vi "MSSQL_Select.vi"(0 "connection reference":T1, 1 "列名数组":string[](array[string]), 3 "排序条件":string, 5 "表名":string, 9 "查询行数":i32, 11 "异常输入":errorcluster, 12 "查询条件":string) -> (4 "connection reference 2":T1, 6 "变体转换后数据":string[][](array[string]), 8 "完整数据":variant[][](array[variant]), 10 "拼接后的sql语句":string, 14 "操作结果":bool, 15 "异常输出":errorcluster)   [LabVIEW 2018]
uses:
  <vilib>/addons/database/Connection.llb/Conn ObjectReference.ctl
  <vilib>/addons/database/Connection.llb/Conn Execute.vi
  <vilib>/addons/database/Recordset.llb/Rec Fetch Recordset Data (R).vi
  <vilib>/addons/database/Recordset.llb/Rec Destroy - Connection.vi
  <vilib>/addons/database/NI_Database_API.lvlib
panel:
  # "select操作\nselect * from tbl_name where 条件 order by \nselect 列1，列2，列3 from tbl_name where 条件 order by \nselect操作\nselect top(1) * from tbl_name where 条件 order by \nselect top(1) 列1，列2，列3 from tbl_name where 条件 order by"
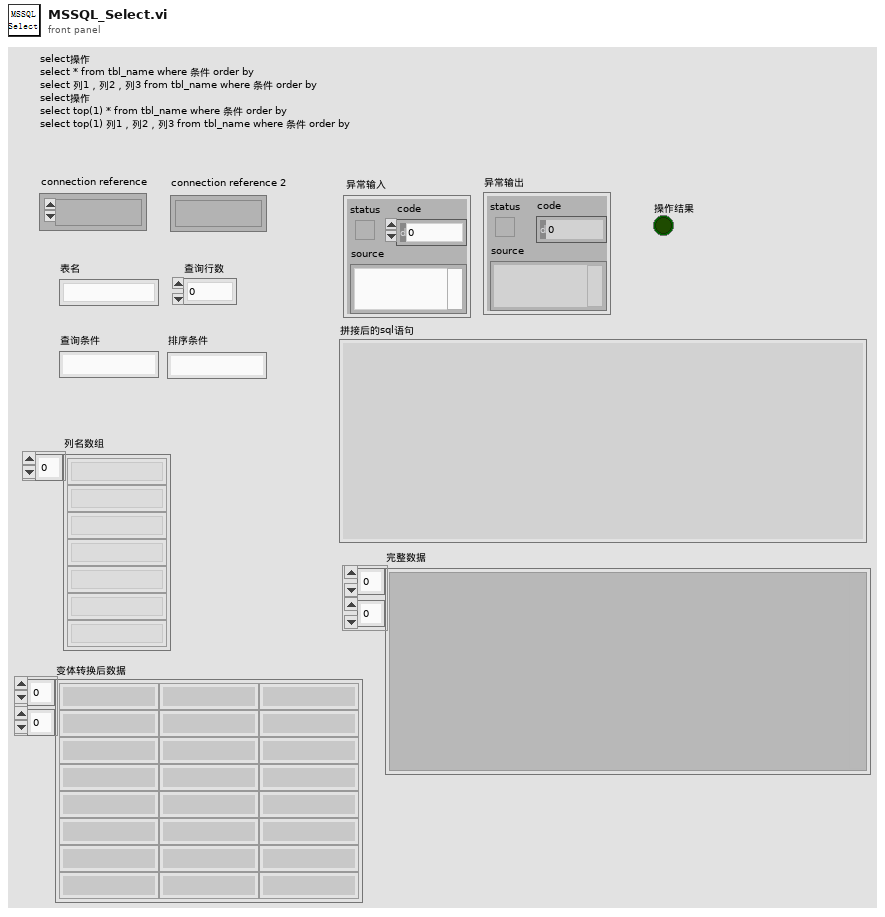
[diagram p1: front panel]
types:
  T1 = typedef "NI_Database_API.lvlib/Conn ObjectReference.ctl" = refnum<k1>
  T2 = typedef "NI_Database_API.lvlib/Rec ObjectReference.ctl" = refnum<k1>
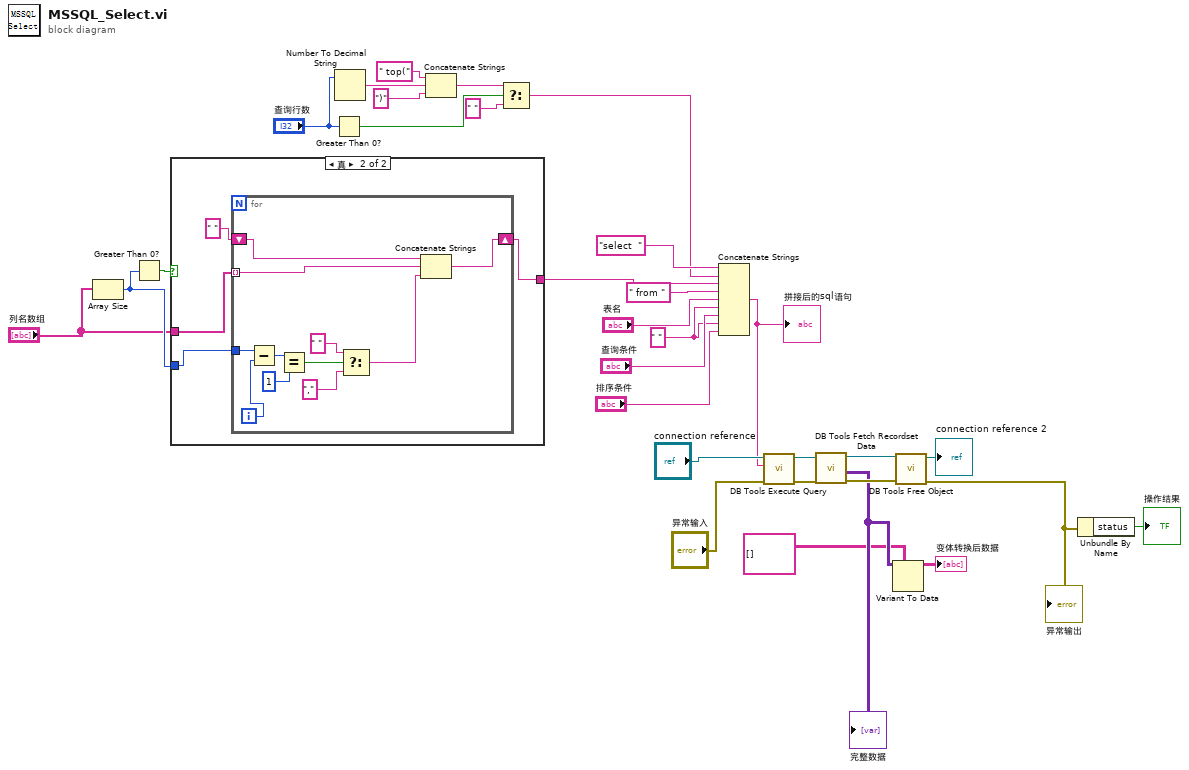
[diagram p0: block diagram]
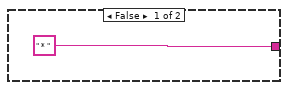
[diagram p2: hidden frame]
diagram:
  w9 = " " ("字符串")
  n1 = Array Size(array="列名数组") -> (size(s)=w29:i32)
  n2 = Greater Than 0?(x=w29) -> (x > 0?=w30:bool)
  n3 = case shown="真" w30 {
    tunnel: [" * " w33] -> w28
    tunnel: w29 -> [_ w36]
    tunnel: "列名数组" -> [_ w35]
    frame False {
    }
    frame True {
      n4 = for {
        tunnel: w35 -> [w46] mode=indexing
        shift-right: [w45] -> w33
        shift-left: " " -> [w47]
        tunnel: w36 -> [w37]
        i -> [w44]
        n5 = Subtract(x=w37, y=w44) -> (x-y=w43:i32)
        n6 = Equal?(x=w43, y=1) -> (x = y?=w41:bool)
        n7 = Select(t=" " ("字符串"), s=w41, f=",") -> (s? t:f=w38:string)
        n8 = Concatenate Strings(w47, w46, w38) -> (w45:string)
      }
    }
  }
  n9 = Greater Than 0?(x="查询行数") -> (x > 0?=w21:bool)
  n10 = Number To Decimal String(number="查询行数") -> (decimal integer string=w16:string)  [unwired: 1 in]
  n11 = Concatenate Strings(" top(" ("字符串"), w16, ")" ("字符串")) -> (w15:string)
  n12 = Select(t=w15, s=w21, f=" ") -> (s? t:f=w14:string)
  n13 = Concatenate Strings("select  ", w14, w28, " from " ("字符串"), "表名", w9, "查询条件", w9, "排序条件") -> (w26:string)
  "拼接后的sql语句" <- w26
  n14 = call-poly <vilib>:"DB Tools Execute Query.vi"("error in (no error)"="异常输入", "SQL query"=w26, "connection reference"="connection reference") -> ("error out"=w6:errorcluster, "recordset reference"=w7:T2)  [unwired: 5 in]
  n15 = call-poly <vilib>:"DB Tools Fetch Recordset Data.vi"("error in (no error)"=w6, "recordset reference"=w7) -> ("error out"=w4:errorcluster, "recordset data"=w3:variant[][], "recordset reference out"=w5:T2)  [unwired: 3 in]
  "完整数据" <- w3
  n16 = Variant To Data(type=string[][] [], Variant=w3) -> (data=→"变体转换后数据":string[][])  [unwired: 1 in, 1 out]
  n17 = call-poly <vilib>:"DB Tools Free Object.vi"("error in (no error)"=w4, "recordset reference"=w5) -> ("error out"=w23:errorcluster, "connection reference"=→"connection reference 2":T1)  [unwired: 8 in]
  "异常输出" <- w23
  n18 = Unbundle By Name(w23) -> ("status"=→"操作结果":bool)
